vi "File_process.vi"() -> ()   [LabVIEW 2023]
uses:
  <vilib>/Utility/file.llb/Read Delimited Spreadsheet (string).vi
  <vilib>/Utility/file.llb/Write Delimited Spreadsheet (string).vi
panel:
  out "Duration time(s)":u32
  out "progress...":u8(slide) scale=0.0..100.0
  in  "stop":bool
  out "offset":dbl
  out "1st row":string[](array[string])
  out "element":i32
  out "size(s)":i32[](array[numeric])
  out "all data":string[][](array[string])
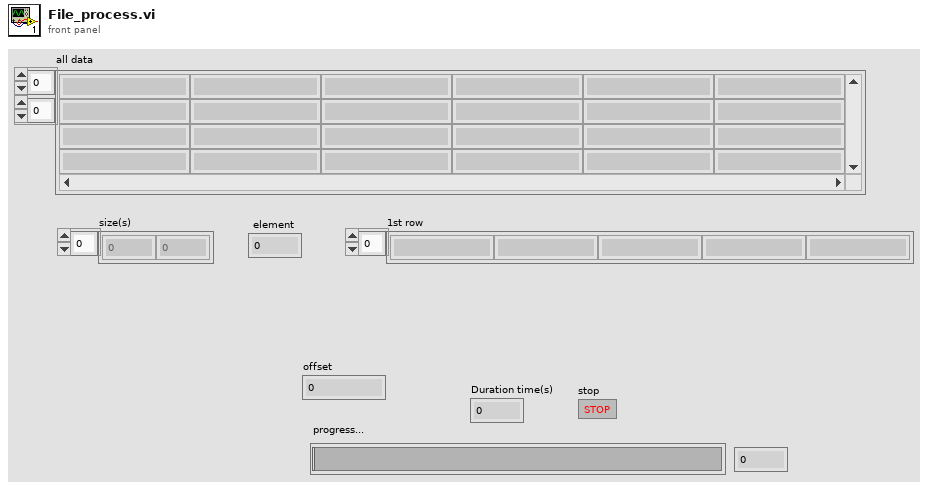
[diagram p1: front panel]
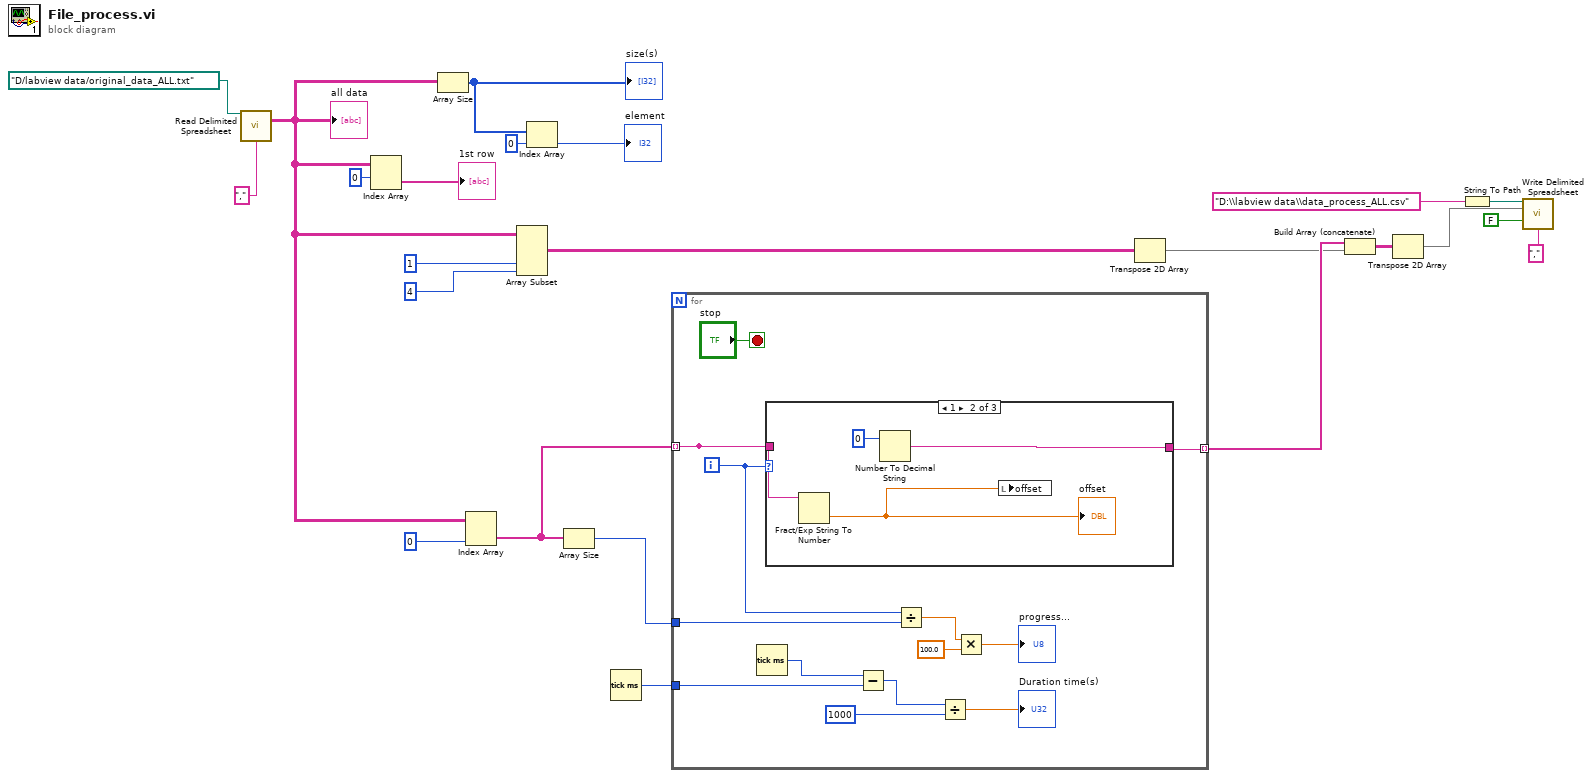
[diagram p0: block diagram]
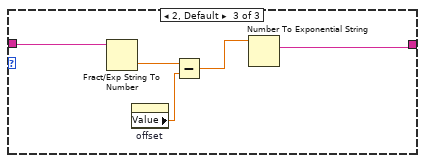
[diagram p3: hidden frame]
diagram:
  n1 = call-poly <vilib>:"Read Delimited Spreadsheet.vi"("file path (dialog if empty)"=path "D:/labview data/original_data_ALL.txt" ("file path (use dialog)"), "delimiter (\\t)"="," ("delimiter (\\t)")) -> ("all rows"=w11:string[][])  [unwired: 8 in, 5 out]
  "all data" <- w11
  n2 = Index Array "Index Array"(array=w11, index (row)=0) -> (element=→"1st row":string[])  [unwired: 1 in]
  n3 = Array Size(array=w11) -> (size(s)=w21:i32[])
  "size(s)" <- w21
  n4 = Index Array(array=w11, index (col)=0 ("index (row)")) -> (element=w13:string[])  [unwired: 1 in]
  n5 = Array Subset "Array Subset"(array=w11, index (col)=1 ("index"), length (col)=4 ("length")) -> (w10:string[][])  [unwired: 2 in]
  n6 = Index Array "Index Array"(array=w21, index=0) -> (element=→"element":i32)
  n7 = Array Size(array=w13) -> (size(s)=w12:i32)
  n8 = Tick Count (ms)() -> (millisecond timer value=w1:u32)
  n9 = for {
    tunnel: w13 -> [w24] mode=indexing
    tunnel: [w36] -> w9 mode=indexing
    tunnel: w12 -> [w33]
    tunnel: w1 -> [w28]
    tunnel: [w24] -> _ mode=indexing
    i -> [w34]
    stop <- "stop" stop-if-true
    n10 = Tick Count (ms)() -> (millisecond timer value=w29:u32)
    n11 = case shown="1" w34 {
      tunnel: w24 -> [w37 w39 w46]
      tunnel: [w37 w40 w43] -> w36
      frame 0 {
      }
      frame 1 {
        n12 = Fract/Exp String To Number(string=w39) -> (number=w38:dbl)  [unwired: 3 in, 1 out]
        "offset" <- w38
        n13 = Number To Decimal String(number=0) -> (decimal integer string=w40:string)  [unwired: 1 in]
        n14 = local write "offset"(w38) -> ()
      }
      frame 2, Default {
        n15 = Fract/Exp String To Number(string=w46) -> (number=w45:dbl)  [unwired: 3 in, 1 out]
        n16 = property on="offset" class="DigNum (strict)"() -> ("Value"=w44:dbl)  [unwired: 2 in, 2 out]
        n17 = Subtract(x=w45, y=w44) -> (x-y=w42:dbl)
        n18 = Number To Exponential String(number=w42) -> (E-format string=w43:string)  [unwired: 3 in]
      }
    }
    n19 = Subtract(x=w29, y=w28) -> (x-y=w27:u32)
    n20 = Divide(x=w34, y=w33) -> (x/y=w32:dbl)
    n21 = Divide(x=w27, y=u32 1000) -> (x/y=→"Duration time(s)":dbl)
    n22 = Multiply(x=w32, y=100.0) -> (x*y=→"progress...":dbl)
  }
  n23 = Transpose 2D Array(2D array=w10) -> (transposed array=w8:string[][])
  n24 = Build Array (concatenate)(w9, w8) -> (w7:string[][])
  n25 = Transpose 2D Array(2D array=w7) -> (transposed array=w2:string[][])
  n26 = String To Path(string="D:\\labview data\\data_process_ALL.csv") -> (path=w4:path)
  n27 = call-poly <vilib>:"Write Delimited Spreadsheet.vi"("file path (dialog if empty)"=w4, "2D data"=w2, "append to file? (new file:F)"=FALSE, "delimiter (\\t)"=",") -> ()  [unwired: 10 in, 2 out]
